vi "SynapseAPI-Set Subject.vi"(0 "URL":string="http://localhost:24414", 7 "subject":string, 11 "error in (no error)":errorcluster) -> (15 "error out":errorcluster)   [LabVIEW 2020]
uses:
  <vilib>/httpClient/PUTBuffer.vi
  <vilib>/httpClient/LabVIEWHTTPClient.lvlib
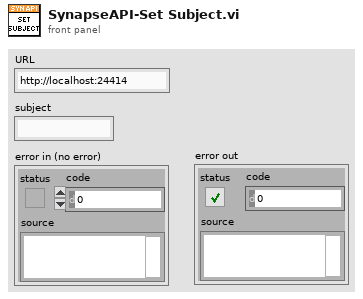
[diagram p1: front panel]
types:
  T1 = typedef "LabVIEWHTTPClient.lvlib/ClientHandle.ctl" = refnum<k1>
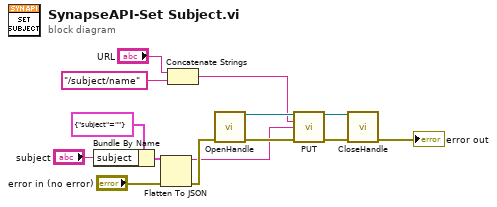
[diagram p0: block diagram]
diagram:
  n1 = Bundle By Name(cluster=cluster{"subject":string} {"subject"=""} ("Cluster"), "subject"="subject") -> (w13:cluster{"subject":string})
  n2 = Flatten To JSON(anything=w13, error in (no error)="error in (no error)") -> (JSON string=w4:string, 11:w5:errorcluster)  [unwired: 1 in]
  n3 = Concatenate Strings("URL", "/subject/name") -> (w6:string)
  n4 = call <vilib>:"OpenHandle.vi"("error in (no error)"=w5) -> ("client handle out"=w9:T1, "error out"=w8:errorcluster)  [unwired: 13 in]
  n5 = call-poly <vilib>:"PUT.vi"("client handle"=w9, "url"=w6, "buffer"=w4, "error in (no error)"=w8) -> ("client handle out"=w11:T1, "error out"=w12:errorcluster)  [unwired: 8 in, 2 out]
  n6 = call <vilib>:"CloseHandle.vi"("client handle"=w11, "error in (no error)"=w12) -> ("error out"=→"error out":errorcluster)  [unwired: 13 in]
